vi "Config-Sweep-Parameters.vi"(7 "delay time (sec)":dbl format="%.4f", 8 "error in (no error)":errorcluster, 9 "hold time (sec)":dbl format="%.4f", 10 "stop condition (free run:0)":u8(ring) items=["continue at any (free run)", "stop at any abnorm", "stop at compliance"], 11 "VISA session":refnum<visa-resource-name>) -> (0 "error out":errorcluster, 3 "VISA resource name out":refnum<visa-resource-name>)   [LabVIEW 2016, in "Agilent 415X Series.lvlib"]
doc: "This VI sets up general parameters for SWEEP mode operation."
uses:
  Agilent 415X Series.lvlib
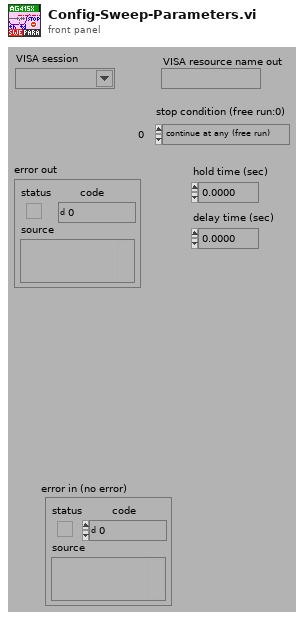
[diagram p1: front panel]
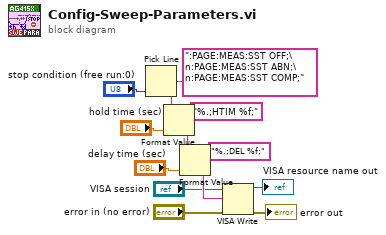
[diagram p0: block diagram]
diagram:
  n1 = Pick Line(multi-line string=":PAGE:MEAS:SST OFF;\n:PAGE:MEAS:SST ABN;\n:PAGE:MEAS:SST COMP;", line index="stop condition (free run:0)") -> (output string=w11:string)  [unwired: 1 in]
  n2 = Format Value(string ("")=w11, format string="%.;HTIM %f;", value (0)="hold time (sec)") -> (output string=w6:string)
  n3 = Format Value(string ("")=w6, format string="%.;DEL %f;", value (0)="delay time (sec)") -> (output string=w3:string)
  n4 = VISA Write(VISA resource name="VISA session", write buffer=w3, error in (no error)="error in (no error)") -> (VISA resource name out=→"VISA resource name out":refnum<visa-resource-name>, error out=→"error out":errorcluster)  [unwired: 1 out]
